vi "WebSocket_Polling.vi"(8 "error in":errorcluster, 11 "WebSocket Connection in":refnum<class "WebSocket Server.lvclass">) -> (0 "error out":errorcluster, 3 "WebSocket Connection out":refnum<class "WebSocket Server.lvclass">, 4 "Boolean":bool)   [LabVIEW 2020]
doc: "For polling the messages from the web page"
uses:
  dependencies/WebSockets-API/Source/WebSockets/WebSocket Server/WebSocket Server.lvclass
  src/user_interfaces/simple_html_chat_ui/typedefs/ui_user_event.ctl
  src/user_interfaces/simple_html_chat_ui/simple_html_chat_ui.lvclass
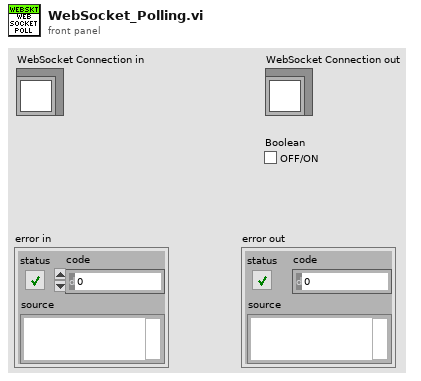
[diagram p1: front panel]
types:
  T1 = typedef "simple_html_chat_ui.lvclass/ui_user_event.ctl" = enum16{"Initialize", "Generate", "Get Reference", "Destroy"}
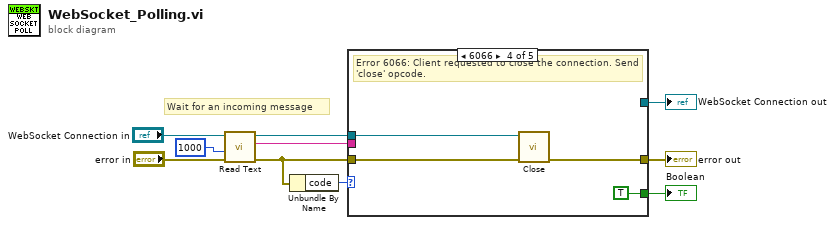
[diagram p0: block diagram]
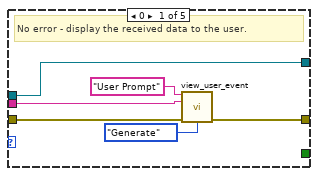
[diagram p2: hidden frame]
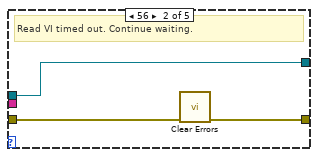
[diagram p3: hidden frame]
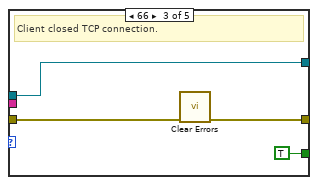
[diagram p4: hidden frame]
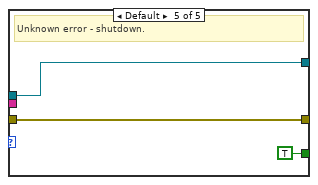
[diagram p5: hidden frame]
diagram:
  # "Wait for an incoming message"
  n1 = call-dynamic "Read Text.vi"("error in (no error)"="error in", "timeout ms (5000)"=1000 ("timeout ms (25000)"), "WebSocket in"="WebSocket Connection in") -> ("error out"=w4:errorcluster, "Data"=w6:string, "WebSocket out"=w5:refnum<class "WebSocket Server.lvclass">)  [unwired: 6 in]
  n2 = Unbundle By Name(w4) -> ("code"=w7:i32)
  n3 = case shown="6066" w7 {
    tunnel: w6 -> [w14 _ _ _ _]
    tunnel: [_ _ TRUE TRUE TRUE] -> w2
    tunnel: w5 -> [w11 w17 w20 w27 w28]
    tunnel: w4 -> [w15 w19 w22 w25 w29]
    tunnel: [w16 w18 w21 w24 w29] -> w3
    tunnel: [w11 w17 w20 _ w28] -> w1
    frame 0 {
      # "No error - display the received data to the user."
      n4 = call "view_user_event.vi"("State"="User Prompt", "Data"=w14, "error in (no error)"=w15, "Operation"=ui_user_event."Generate") -> ("error out"=w16:errorcluster)  [unwired: 10 in, 1 out]
    }
    frame 56 {
      # "Read VI timed out. Continue waiting."
      n5 = call <vilib>:"Clear Errors.vi"("error in (no error)"=w19) -> ("error out"=w18:errorcluster)  [unwired: 5 in, 1 out]
    }
    frame 66 {
      # "Client closed TCP connection."
      n6 = call <vilib>:"Clear Errors.vi"("error in (no error)"=w22) -> ("error out"=w21:errorcluster)  [unwired: 5 in, 1 out]
    }
    frame 6066 {
      # "Error 6066: Client requested to close the connection. Send 'close' opcode."
      n7 = call-dynamic "Close.vi"("error in (no error)"=w25, "WebSocket in"=w27) -> ("error out"=w24:errorcluster)  [unwired: 9 in]
    }
    frame Default {
      # "Unknown error - shutdown."
    }
  }
  "error out" <- w3
  "Boolean" <- w2
  "WebSocket Connection out" <- w1
